vi "Write Path.vi"(8 "error in (no error)":errorcluster, 10 "Path":path, 11 "Login bin in":refnum<class "Login bin.lvclass">) -> (0 "error out":errorcluster, 3 "Login bin out":refnum<class "Login bin.lvclass">)   [LabVIEW 2020, in "Login bin.lvlib" / "Login bin.lvclass"]
uses:
  Login bin.lvclass
  Login bin.lvclass/Login bin.ctl
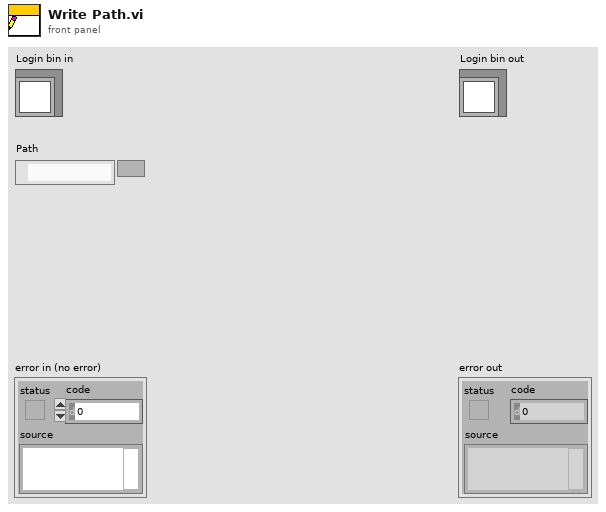
[diagram p1: front panel]
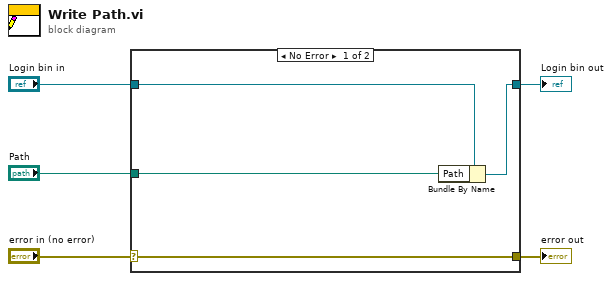
[diagram p0: block diagram]
diagram:
  n1 = case shown="No Error" "error in (no error)" {
    selector: "error in (no error)" -> [w9 w10]
    tunnel: [w9 w10] -> w4
    tunnel: [w7 w11] -> w2
    tunnel: "Login bin in" -> [w8 w11]
    tunnel: "Path" -> [w6 _]
    frame No Error {
      n2 = Bundle By Name(cluster=w8, "Path"=w6) -> (w7:refnum<class "Login bin.lvclass">)
    }
    frame Error {
    }
  }
  "error out" <- w4
  "Login bin out" <- w2
